vi "[RT]Read_TC_Temp2.vi"(8 "error in (no error)":errorcluster, 11 "Stop":bool=TRUE) -> (0 "error out":errorcluster, 3 "TEC Temp [°C]":dbl)   [LabVIEW 2018]
uses:
  <vilib>/myRIO/Instrument Drivers/Onboard IO/SPI/typedefs/SPI User Configuration.ctl
  <vilib>/myRIO/Common/Instrument Driver Framework/myRIO v1.0/SPI/typedefs/SPI Clock Phase.ctl
  <vilib>/myRIO/Common/Instrument Driver Framework/myRIO v1.0/SPI/typedefs/SPI Clock Polarity.ctl
  <vilib>/myRIO/Common/Instrument Driver Framework/myRIO v1.0/SPI/typedefs/SPI Data Direction.ctl
  <vilib>/myRIO/Common/Instrument Driver Framework/myRIO v1.0/SPI/typedefs/SPI Frame Length.ctl
  <vilib>/myRIO/Instrument Drivers/Onboard IO/SPI/typedefs/SPI Reference.ctl
  <vilib>/myRIO/Common/Instrument Driver Framework/Utilities/typedefs/myRIO Generic Hardware Reference.ctl
  <vilib>/myRIO/Common/Instrument Driver Framework/Utilities/typedefs/Hardware Version Enum.ctl
  <vilib>/myRIO/Common/Instrument Driver Framework/Utilities/typedefs/myRIO v1.0 Reference.ctl
  <vilib>/myRIO/Common/Instrument Driver Framework/Utilities/typedefs/Generic FPGA Reference.ctl
  <vilib>/myRIO/Common/Instrument Driver Framework/myRIO v1.0/SPI/typedefs/SPI Channels Enum.ctl
  <vilib>/myRIO/Instrument Drivers/Onboard IO/SPI/typedefs/SPI Configuration.ctl
  <vilib>/userdefined/High Color/nirio_resource_hc.ctl
  <vilib>/myRIO/Instrument Drivers/Onboard IO/DIO/typedefs/DIO Reference.ctl
  <vilib>/myRIO/Common/Instrument Driver Framework/myRIO v1.0/DIO/typedefs/DIO Channels List.ctl
  <vilib>/myRIO/Common/Instrument Driver Framework/myRIO v1.0/DIO/typedefs/DIO Channels Enum.ctl
  <vilib>/myRIO/Common/Instrument Driver Framework/myRIO v1.0/SPI/vis/myRIO v1.1 Open SPI.vi
  <vilib>/myRIO/Common/Instrument Driver Framework/myRIO v1.0/DIO/vis/myRIO v1.1 Open DIO.vi
  <vilib>/myRIO/Common/Instrument Driver Framework/Utilities/vis/Validate Channels.vi
  <vilib>/myRIO/Common/Instrument Driver Framework/myRIO v1.0/SPI/vis/myRIO v1.0 Reserve SPI.vi
  <vilib>/myRIO/Common/Instrument Driver Framework/myRIO v1.0/DIO/vis/myRIO v1.0 Reserve DIO.vi
  <vilib>/myRIO/Instrument Drivers/Onboard IO/SPI/vis/Write Read.vi
  <vilib>/myRIO/Common/Instrument Driver Framework/myRIO v1.0/DIO/vis/myRIO v1.0 Close DIO.vi
  <vilib>/myRIO/Common/Instrument Driver Framework/myRIO v1.0/SPI/vis/myRIO v1.0 Close SPI.vi
  <vilib>/myRIO/Common/Instrument Driver Framework/myRIO v1.0/SPI/vis/myRIO v1.0 Build MUX Configuration SPI.vi
  <vilib>/myRIO/Common/Instrument Driver Framework/myRIO v1.0/Resource Manager/vis/myRIO v1.0 Reserve Channel List.vi
  <vilib>/myRIO/Common/Instrument Driver Framework/myRIO v1.0/DIO/vis/myRIO v1.0 Build MUX Configuration DIO.vi
  <vilib>/myRIO/Common/Instrument Driver Framework/myRIO v1.0/DIO/vis/myRIO v1.0 Unreserve DIO.vi
  <vilib>/myRIO/Common/Instrument Driver Framework/myRIO v1.0/SPI/vis/myRIO v1.0 Unreserve SPI.vi
  <vilib>/myRIO/Common/Instrument Driver Framework/myRIO v1.0/Resource Manager/vis/myRIO v1.0 Create Configuration List.vi
  <vilib>/myRIO/Common/Instrument Driver Framework/myRIO v1.0/Resource Manager/vis/myRIO v1.0 Reserve Channel.vi
  <vilib>/myRIO/Common/Instrument Driver Framework/myRIO v1.0/Resource Manager/vis/myRIO v1.0 Unreserve Channel.vi
  <vilib>/myRIO/Common/Instrument Driver Framework/myRIO v1.0/Resource Manager/vis/myRIO v1.0 Unreserve Channel List.vi
  <vilib>/myRIO/Common/Instrument Driver Framework/myRIO v1.0/Resource Manager/vis/myRIO v1.0 Build Mutex Name.vi
  <vilib>/Utility/VariantDataType/GetNumericInfo.vi
  <vilib>/Utility/error.llb/Error Cluster From Error Code.vi
  <vilib>/myRIO/Common/Instrument Driver Framework/myRIO v1.0/myRIO v1.1 Open.vi
  <vilib>/myRIO/Common/Instrument Driver Framework/Utilities/vis/IO Manager.vi
  <vilib>/myRIO/Common/Instrument Driver Framework/Utilities/vis/Configuration Manager.vi
  <vilib>/myRIO/Common/Instrument Driver Framework/myRIO v1.0/Resource Manager/vis/myRIO v1.0 Configure IO.vi
  <vilib>/myRIO/Common/Instrument Driver Framework/myRIO v1.0/myRIO v1.0 Close.vi
  <vilib>/myRIO/Common/Instrument Driver Framework/myRIO v1.0/SPI/vis/myRIO v1.0 Configure SPI.vi
  <vilib>/myRIO/Common/Instrument Driver Framework/myRIO v1.0/DIO/vis/myRIO v1.0 Write DIO.vi
  [GlobVar]SensorState.vi
  [GlobVar]Param.vi
  <vilib>/myRIO/Common/Instrument Driver Framework/myRIO v1.0/SPI/vis/myRIO v1.0 Write Read SPI.vi
  <vilib>/myRIO/Common/Instrument Driver Framework/myRIO v1.0/DIO/vis/myRIO v1.0 Shutdown DIO.vi
  <vilib>/myRIO/Common/Instrument Driver Framework/myRIO v1.0/SPI/vis/myRIO v1.0 Shutdown SPI.vi
  <vilib>/myRIO/Instrument Drivers/Onboard IO/SPI/vis/myRIO SPI Open.xnode
  <vilib>/myRIO/Instrument Drivers/Onboard IO/DIO/vis/myRIO DIO Open.xnode
  <vilib>/myRIO/Instrument Drivers/Onboard IO/SPI/SPI.lvlib
  <vilib>/myRIO/Instrument Drivers/Onboard IO/DIO/DIO.lvlib
panel:
  in  "Stop 2":bool=TRUE
  out "Frames Read":u16[](array[numeric])
  out "CJC Temp [°C]":dbl
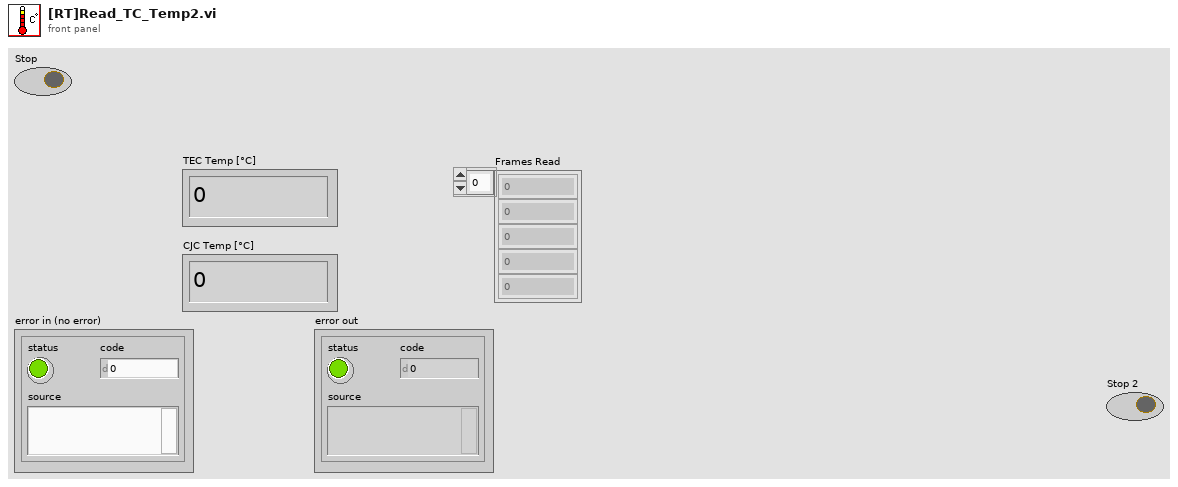
[diagram p1: front panel]
types:
  T1 = enum16{"Close Readubg", "Read", "Enable Reading", "Error Handling"}
  T2 = typedef "SPI.lvlib/SPI User Configuration.ctl" = cluster{"Frequency [Hz]":dbl, "Clock Phase":T3, "Clock Polarity":T4, "Data Direction":T5, "Frame Length":T6}
  T3 = typedef "SPI Clock Phase.ctl" = enum8{"Leading", "Trailing"}
  T4 = typedef "SPI Clock Polarity.ctl" = enum8{"Low", "High"}
  T5 = typedef "SPI Data Direction.ctl" = enum8{"Most significant bit first", "Least significant bit first"}
  T6 = typedef "SPI Frame Length.ctl" = u8
  T7 = typedef "DIO.lvlib/DIO Reference.ctl" = cluster{"myRIO Reference":T8, "DIO Channels List":T12}
  T8 = typedef "myRIO Generic Hardware Reference.ctl" = cluster{"myRIO Model":T9, "myRIO Hardware Reference":T10}
  T9 = typedef "Hardware Version Enum.ctl" = enum16{"Unknown", "myRIO-1900", "myRIO-1950", "roboRIO", "NI ELVIS RIO CM", "ELVIS III"}
  T10 = typedef "myRIO v1.0 Reference.ctl" = cluster{"Generic FPGA Reference":T11, "Allow multiple opens":bool}
  T11 = typedef "Generic FPGA Reference.ctl" = refnum<k20>
  T12 = typedef "DIO Channels List.ctl" = T13[]
  T13 = typedef "DIO Channels Enum.ctl" = enum16{"Not Connected", "C/DIO0", "C/DIO1", "C/DIO2", "C/DIO3", "C/DIO4", "C/DIO5", "C/DIO6", "C/DIO7", "A/DIO0", "A/DIO1", "A/DIO2", "A/DIO3", "A/DIO4", "A/DIO5", "A/DIO6", "A/DIO7", "A/DIO8", "A/DIO9", "A/DIO10", "A/DIO11", "A/DIO12", "A/DIO13", "A/DIO14", "A/DIO15", "A/DIO16", "A/DIO17", "A/DIO18", "A/DIO19", "B/DIO0", "B/DIO1", "B/DIO2", "B/DIO3", "B/DIO4", "B/DIO5", "B/DIO6", "B/DIO7", "B/DIO8", "B/DIO9", "B/DIO10", "B/DIO11", "B/DIO12", "B/DIO13", "B/DIO14", "B/DIO15", "B/DIO16", "B/DIO17", "B/DIO18", "B/DIO19", "LED0", "LED1", "LED2", "LED3", "Button0", "DIO/DIO0", "DIO/DIO1", "DIO/DIO2", "DIO/DIO3", "DIO/DIO4", "DIO/DIO5", "DIO/DIO6", "DIO/DIO7", "DIO/DIO8", "DIO/DIO9", "SPI/CS0", "SPI/CS1", "SPI/CS2", "SPI/CS3", "LED RADIO (Green)", "LED RADIO (Red)", "LED COMM (Green)", "LED COMM (Red)", "LED MODE (Green)", "LED MODE (Red)"}
  T14 = typedef "SPI.lvlib/SPI Reference.ctl" = cluster{"myRIO Reference":T8, "SPI Channels Enum":T15, "SPI Configuration":T16}
  T15 = typedef "SPI Channels Enum.ctl" = enum16{"Not Connected", "A/SPI", "B/SPI", "SPI/SPI"}
  T16 = typedef "SPI.lvlib/SPI Configuration.ctl" = cluster{"Frequency [Hz]":dbl, "Clock Phase":T3, "Clock Polarity":T4, "Data Direction":T5, "Frame Length":T6}
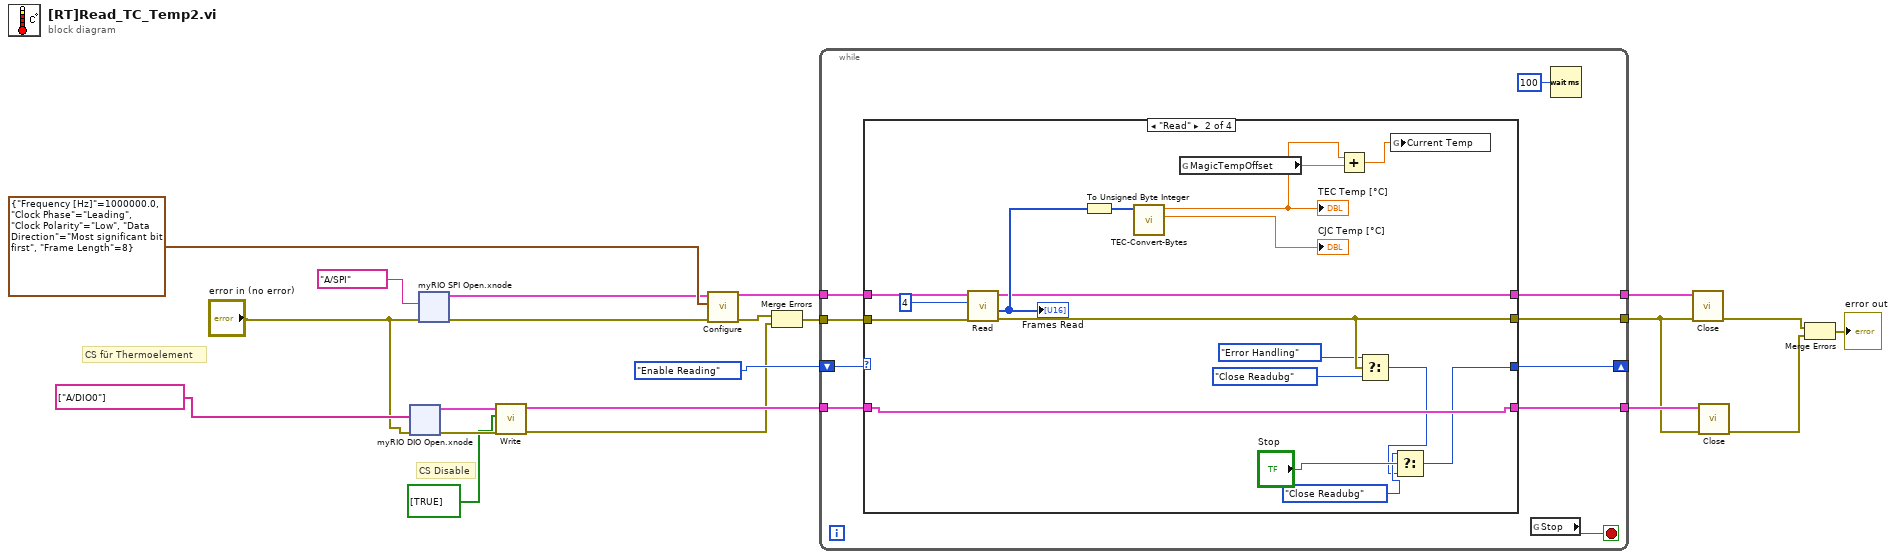
[diagram p0: block diagram]
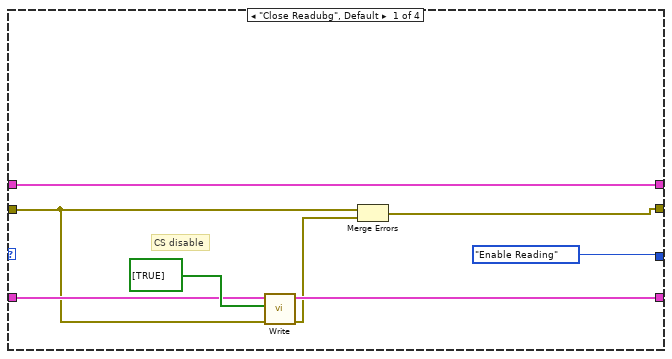
[diagram p2: hidden frame]
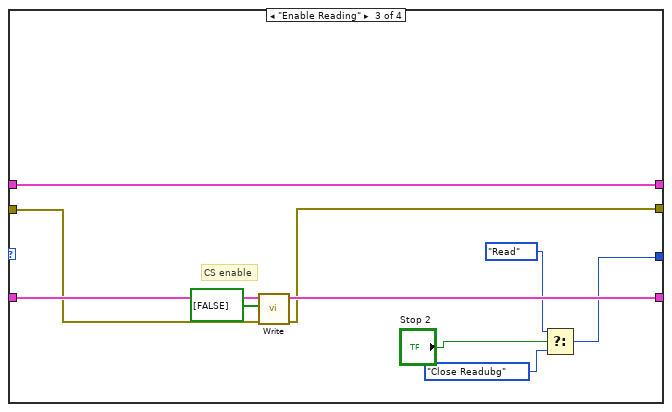
[diagram p3: hidden frame]
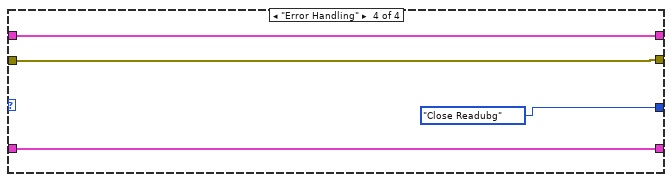
[diagram p4: hidden frame]
diagram:
  # "CS Disable"
  # "CS für Thermoelement"
  n1 = xnode "myRIO DIO Open.xnode"("error in (no error)"="error in (no error)", "Channel Names"=tag[] ["A/DIO0"]) -> ("error out"=w13:errorcluster, "DIO Ref Out"=w15:T7)  [unwired: 1 in]
  n2 = xnode "myRIO SPI Open.xnode"("error in (no error)"="error in (no error)", "Channel Name"=tag "A/SPI") -> ("error out"=w17:errorcluster, "SPI Ref Out"=w16:T14)  [unwired: 1 in]
  n3 = call <vilib>:"Write.vi"("error in (no error)"=w13, "Values"=bool[] [TRUE], "DIO Ref In"=w15) -> ("error out"=w7:errorcluster, "DIO Ref Out"=w9:T7)  [unwired: 6 in]
  n4 = call <vilib>:"Configure.vi"("error in (no error)"=w17, "SPI User Configuration"=T2 {"Frequency [Hz]"=1000000.0, "Clock Phase"=enum."Leading", "Clock Polarity"=enum."Low", "Data Direction"=enum."Most significant bit first", "Frame Length"=8}, "SPI Ref In"=w16) -> ("error out"=w6:errorcluster, "SPI Ref Out"=w20:T14)  [unwired: 7 in]
  n5 = Merge Errors(w6, w7) -> (w5:errorcluster)
  n6 = while {
    tunnel: w5 -> [w31]
    tunnel: w20 -> [w30]
    tunnel: [w28] -> w19
    tunnel: [w27] -> w8
    shift-right: [w23] -> _
    shift-left: T1."Enable Reading" -> [w26]
    tunnel: [w25] -> w10
    tunnel: w9 -> [w24]
    stop <- w22 stop-if-true
    n7 = case shown="\"Read\"" w26 {
      tunnel: w31 -> [w35 w56 w64 w70]
      tunnel: w30 -> [w33 w55 w62 w71]
      tunnel: [w33 w51 w62 w71] -> w28
      tunnel: [w34 w49 w63 w70] -> w27
      tunnel: [w39 w50 w67 w68] -> w25
      tunnel: w24 -> [w37 w50 w66 w68]
      tunnel: [T1."Enable Reading" w45 w58 T1."Close Readubg"] -> w23
      frame "Close Readubg", Default {
        # "CS disable"
        n8 = call <vilib>:"Write.vi"("error in (no error)"=w35, "Values"=bool[] [TRUE], "DIO Ref In"=w37) -> ("error out"=w36:errorcluster, "DIO Ref Out"=w39:T7)  [unwired: 6 in]
        n9 = Merge Errors(w35, w36) -> (w34:errorcluster)
      }
      frame "Read" {
        n10 = call <vilib>:"Read.vi"("error in (no error)"=w56, "Frame Count"=u32 4, "SPI Ref In"=w55) -> ("error out"=w49:errorcluster, "Frames Read"=w53:u16[], "SPI Ref Out"=w51:T14)  [unwired: 5 in]
        "Frames Read" <- w53
        n11 = To Unsigned Byte Integer(number=w53) -> (unsigned 8bit integer=w54:u8[])
        n12 = call "TEC-Convert-Bytes.vi"("Frames Read"=w54) -> ("CJC Temp [°C]"=→"CJC Temp [°C]":dbl, "TEC Temp [°C]"=w42:dbl)  [unwired: 5 in, 4 out]
        "TEC Temp [°C]" <- w42
        n13 = global read "[GlobVar]Param.vi" "MagicTempOffset"() -> (w41:dbl)
        n14 = Add(x=w42, y=w41) -> (x+y=w40:dbl)
        n15 = Select(t=T1."Error Handling", s=w49, f=T1."Close Readubg") -> (s? t:f=w43:T1)
        n16 = global write "[GlobVar]SensorState.vi" "Current Temp"(w40) -> ()
        n17 = Select(t=T1."Close Readubg", s="Stop", f=w43) -> (s? t:f=w45:T1)
      }
      frame "Enable Reading" {
        # "CS enable"
        n18 = call <vilib>:"Write.vi"("error in (no error)"=w64, "Values"=bool[] [FALSE], "DIO Ref In"=w66) -> ("error out"=w63:errorcluster, "DIO Ref Out"=w67:T7)  [unwired: 6 in]
        n19 = Select(t=T1."Read", s="Stop 2", f=T1."Close Readubg") -> (s? t:f=w58:T1)
      }
      frame "Error Handling" {
      }
    }
    n20 = global read "[GlobVar]SensorState.vi" "Stop"() -> (w22:bool)
    n21 = Wait (ms)(milliseconds to wait=u32 100) -> ()  [unwired: 1 out]
  }
  n22 = call <vilib>:"Close.vi"("error in (no error)"=w8, "SPI Ref In"=w19) -> ("error out"=w3:errorcluster)  [unwired: 9 in]
  n23 = call <vilib>:"Close.vi"("error in (no error)"=w8, "DIO Ref In"=w10) -> ("error out"=w2:errorcluster)  [unwired: 9 in]
  n24 = Merge Errors(w3, w2) -> (→"error out":errorcluster)
